vi "FindAvailableIP.vi"(0 "IP Address":string="0.0.0.0", 1 "Subnet Mask":string="255.255.255.255") -> (3 "bit Mask":string="/32", 4 "Highest usable address":string="0.0.0.0", 5 "Lowest usable address":string="0.0.0.0", 6 "Status Table":string[][](table) caption="Address List")   [LabVIEW 2013]
doc: "When adding a device to a network, you must often choose an IP address for the device. The method you use to obtain an IP address may depend on whether you have a network with an administrator or not. If you have a network with an administrator, it is best to consult with the administrator to choose an appropriate IP address for the device. If your network does not have an administrator, or it is necessary to find an available address on your own, you can use this VI to determine which IP addresses on a subnet are available for use. This example automates the task of sequentially pinging multiple IP addresses on a given subnet to determine which IP addresses are available. The pinged IP addresses are added to a table along with their availibility status."
panel:
  out "Currently Pinging:":string
  in  "stop":bool
  # "Overview:  This example automates the task of sequentially pinging multiple IP addresses on a given subnet to determine which IP addresses are available.\n\nRequirements: LabVIEW 2012 (or compatible)\n\nInstructions:\n1. Enter an IP Address that resides\non the subnet you wish to search.\n\n2. Enter the subnet mask for the \nsubnet. \n\n3. Run the VI.\n\n4. Status Table will be updated \nwith the pinged IP addresses and\ntheir availability."
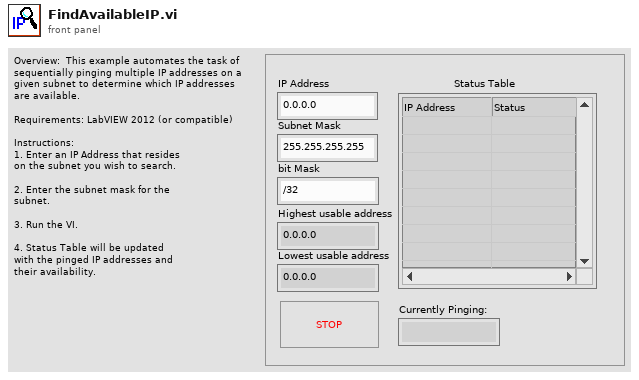
[diagram p1: front panel]
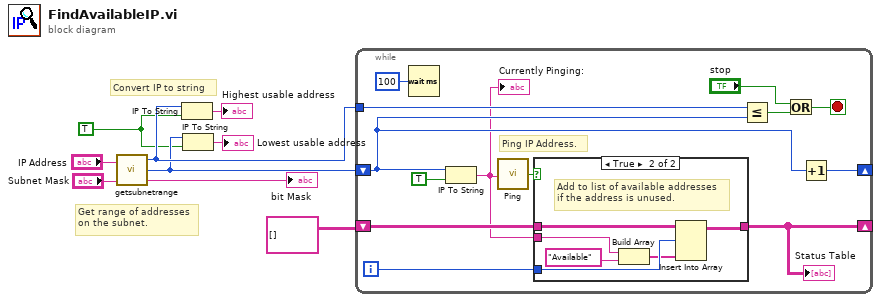
[diagram p0: block diagram]
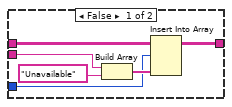
[diagram p2: hidden frame]
diagram:
  w2 = TRUE ("dot notation? (F)")
  # "Convert IP to string"
  # "Get range of addresses\non the subnet."
  n1 = call "getsubnetrange.vi"("IP Address"="IP Address", "Subnet Mask"="Subnet Mask") -> ("Highest Usable Address"=w6:u32, "Lowest Usable Address"=w5:u32, "bit Mask"=→"bit Mask":string)
  n2 = IP To String(1:w2, 2:w6) -> (0:→"Highest usable address":string)
  n3 = IP To String(1:w2, 2:w5) -> (0:→"Lowest usable address":string)
  n4 = while {
    shift-right: [w20] -> _
    shift-left: w5 -> [w19]
    tunnel: w6 -> [w21]
    shift-right: [w17] -> _
    shift-left: string[][] [] -> [w18]
    i -> [w14]
    stop <- w10 stop-if-true
    # "Ping IP Address."
    n5 = Wait (ms)(milliseconds to wait=u32 100) -> ()  [unwired: 1 out]
    n6 = IP To String(1:TRUE ("dot notation? (F)"), 2:w19) -> (0:w16:string)
    "Currently Pinging:" <- w16
    n7 = call "Ping.vi"("PC Name or IP Address"=w16) -> ("Available"=w22:bool)
    n8 = case shown="True" w22 {
      tunnel: w18 -> [w24 w34]
      tunnel: [w23 w29] -> w17
      tunnel: w16 -> [w25 w32]
      tunnel: w14 -> [w26 w33]
      frame False {
        n9 = Build Array(w25, "Unavailable" ("element")) -> (w27:string[])
        n10 = Insert Into Array(array=w24, index (row)=w26, new element=w27) -> (w23:string[][])  [unwired: 1 in]
      }
      frame True {
        # "Add to list of available addresses\nif the address is unused."
        n11 = Build Array(w32, "Available" ("element")) -> (w30:string[])
        n12 = Insert Into Array(array=w34, index (row)=w33, new element=w30) -> (w29:string[][])  [unwired: 1 in]
      }
    }
    "Status Table" <- w17
    n13 = Less Or Equal?(x=w21, y=w19) -> (x <= y?=w12:bool)
    n14 = Or(x="stop", y=w12) -> (x .or. y?=w10:bool)
    n15 = Increment(x=w19) -> (x+1=w20:u32)
  }
